vi "Main For Loop Without Swaps.vi"(0 "A":u32, 1 "80 32-bit Words":u32[](array[numeric]), 5 "B":u32, 7 "C":u32, 9 "D":u32, 11 "E":u32) -> (4 "A Out":u32, 6 "B Out":u32, 8 "C Out":u32, 10 "D Out":u32, 15 "E Out":u32)   [LabVIEW 2014]
uses:
  <vilib>/Platform/TimedLoop/XDataNode/timing_clust.ctl
  <vilib>/Platform/TimedLoop/XDataNode/nitl_modes.ctl
  <vilib>/Platform/TimedLoop/XDataNode/wakeup.ctl
  <vilib>/rvi/Emulation/niFpgaSctlEmulationGetInTimedLoop.vi
  <vilib>/rvi/Emulation/niFpgaEmulationReportErrorSimple.vi
  <vilib>/rvi/Emulation/niFpgaGetClockAttributes.vi
  <vilib>/rvi/Emulation/niFpgaCriticalErrorInLSC.vi
  <vilib>/platform/TimedLoop/XDataNode/XDataNode.xnode
  <vilib>/Platform/TimedLoop/XDataNode/XDNodeRunTimeDep.lvlib
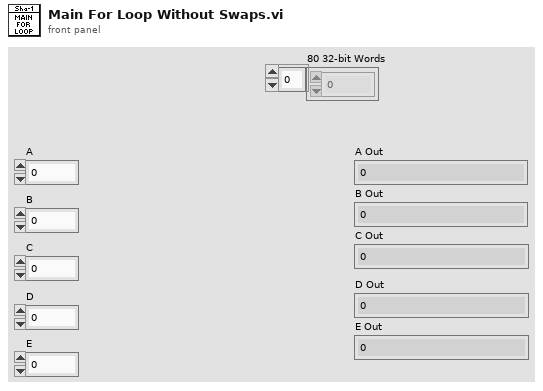
[diagram p1: front panel]
types:
  T1 = typedef "XDNodeRunTimeDep.lvlib/timing_clust.ctl" = cluster{"Expected End [f-1]":u64, "Actual End [f-1]":u64, "Finished Late? [f-1]":bool, "Expected End [i-1]":u64, "Actual End [i-1]":u64, "Finished Late? [i-1]":bool, "Expected Start [i]":u64, "Actual Start [i]":u64, "Expected Start [f]":u64, "Actual Start [f]":u64, "Source Name":string, "Structure Name":string, "Period":i64, "Deadline":i64, "Offset":i64, "Start":i64, "Priority":i32, "Timeout":i32, "Mode":T2, "Wakeup Reason":T3, "Error":errorcluster, "Source Type":string, "Secondary Source Type":string, "Global End Time":u64, "Global Start Time":u64, "Frame Duration":u64, "Iteration Duration":u64, "Assigned CPU":i32, "I/O Scan Engine Mode":u32}
  T2 = typedef "XDNodeRunTimeDep.lvlib/nitl_modes.ctl" = enum32{"No Change", "Process missed periods, maintain original phase", "Discard missed periods, maintain original phase", "Process missed periods, ignore original phase", "Discard missed periods, ignore original phase"}
  T3 = typedef "XDNodeRunTimeDep.lvlib/wakeup.ctl" = enum32{"Normal", "Aborted", "Asynchronous wakeup", "Timing source error", "Timed loop error", "Timeout"}
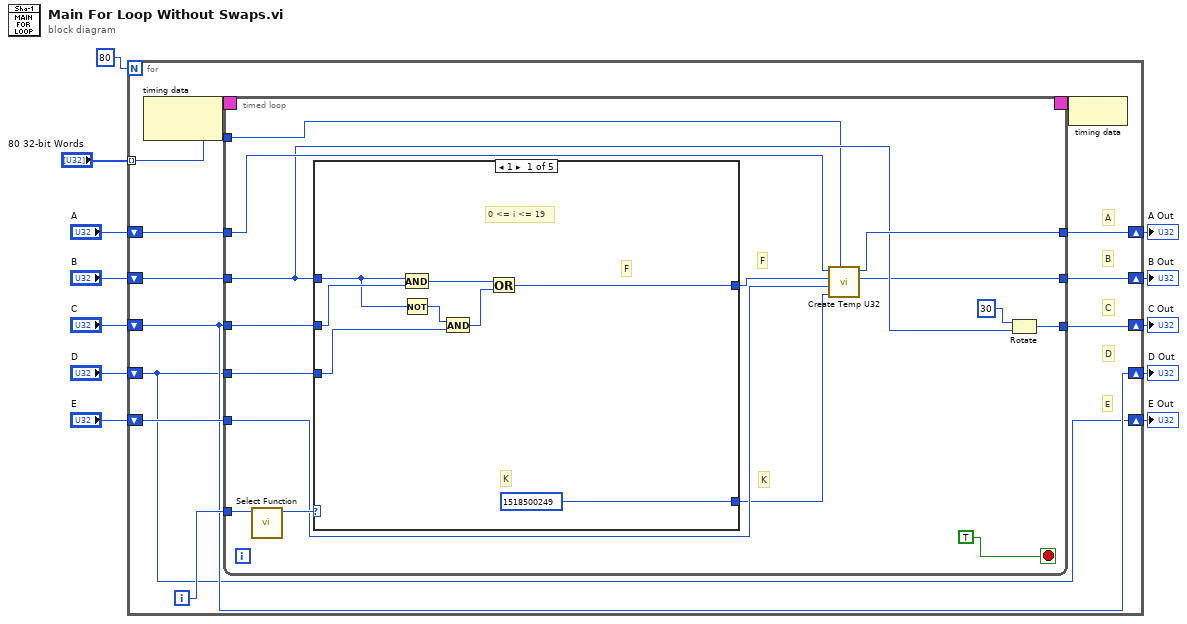
[diagram p0: block diagram]
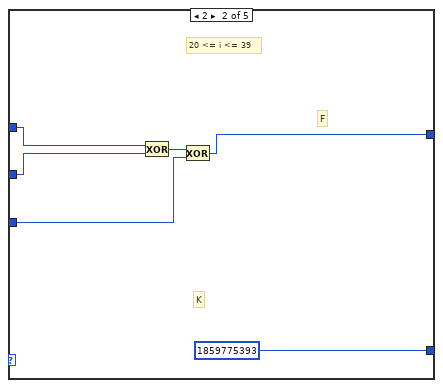
[diagram p2: hidden frame]
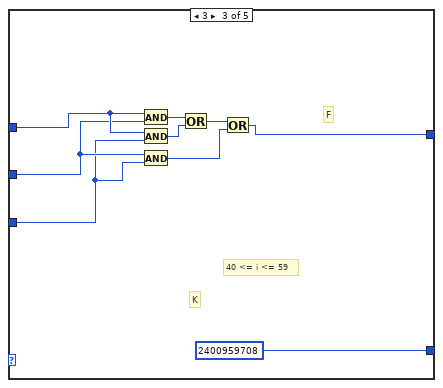
[diagram p3: hidden frame]
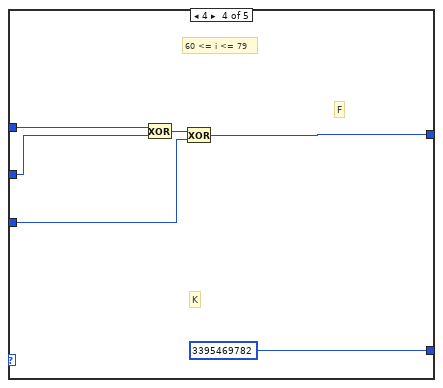
[diagram p4: hidden frame]
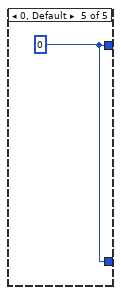
[diagram p5: hidden frame]
diagram:
  n1 = for {
    N: 80 -> [_]
    shift-right: [w21] -> w11
    shift-left: "A" -> [w23]
    shift-right: [w18] -> w10
    shift-left: "B" -> [w20]
    shift-right: [w19] -> w9
    shift-left: "C" -> [w17]
    shift-right: [w17] -> w8
    shift-left: "D" -> [w16]
    shift-right: [w16] -> w7
    shift-left: "E" -> [w22]
    tunnel: "80 32-bit Words" -> [w15] mode=indexing
    i -> [w24]
    # "E"
    # "D"
    # "C"
    # "B"
    # "A"
    n2 = node-c288() -> (w14:T1)  [unwired: 1 in]
    n3 = timed-loop {
      timing: w14 -> [_]
      timing-out: [_] -> w13
      tunnel: w24 -> [w39]
      tunnel: w23 -> [w37]
      tunnel: w22 -> [w35]
      tunnel: [w33] -> w21
      tunnel: w20 -> [w31]
      tunnel: [w30] -> w19
      tunnel: [w29] -> w18
      tunnel: w17 -> [w28]
      tunnel: w16 -> [w27]
      tunnel: w15 -> [w26]
      stop <- TRUE stop-if-true
      # "K"
      # "F"
      n4 = call "Select Function.vi"("Numeric"=w39) -> ("result"=w38:i32)  [unwired: 10 in]
      n5 = case shown="1" w38 {
        tunnel: [u32 1518500249 u32 1859775393 u32 2400959708 u32 3395469782 w69] -> w34
        tunnel: w31 -> [w42 w51 w57 w66 _]
        tunnel: w28 -> [w43 w50 w56 w65 _]
        tunnel: w27 -> [w41 w49 w55 w64 _]
        tunnel: [w40 w48 w54 w63 w69] -> w36
        frame 1 {
          # "F"
          # "0 <= i <= 19"
          # "K"
          n6 = And(x=w42, y=w43) -> (x .and. y?=w46:u32)
          n7 = Not(x=w42) -> (.not. x?=w47:u32)
          n8 = And(x=w47, y=w41) -> (x .and. y?=w45:u32)
          n9 = Or(x=w46, y=w45) -> (x .or. y?=w40:u32)
        }
        frame 2 {
          # "F"
          # "20 <= i <= 39"
          # "K"
          n10 = Exclusive Or(1:w50, 2:w51) -> (0:w53:u32)
          n11 = Exclusive Or(1:w49, 2:w53) -> (0:w48:u32)
        }
        frame 3 {
          # "F"
          # "K"
          # "40 <= i <= 59"
          n12 = And(x=w57, y=w56) -> (x .and. y?=w62:u32)
          n13 = And(x=w57, y=w55) -> (x .and. y?=w61:u32)
          n14 = And(x=w56, y=w55) -> (x .and. y?=w59:u32)
          n15 = Or(x=w62, y=w61) -> (x .or. y?=w60:u32)
          n16 = Or(x=w60, y=w59) -> (x .or. y?=w54:u32)
        }
        frame 4 {
          # "F"
          # "K"
          # "60 <= i <= 79"
          n17 = Exclusive Or(1:w65, 2:w66) -> (0:w68:u32)
          n18 = Exclusive Or(1:w64, 2:w68) -> (0:w63:u32)
        }
        frame 0, Default {
          w69 = u32 0
        }
      }
      n19 = call "Create Temp U32.vi"("W[i]"=w26, "K"=w34, "E"=w35, "F"=w36, "A"=w37) -> ("A Out"=w29:u32, "Temp Out"=w33:u32)  [unwired: 5 in]
      n20 = Rotate(1:w31, 2:i16 30 ("y")) -> (0:w30:u32)
    }
    n21 = node-c288(w13) -> ()
  }
  "A Out" <- w11
  "B Out" <- w10
  "C Out" <- w9
  "D Out" <- w8
  "E Out" <- w7
